vi "Manage logger file txt.vi"(0 "length":i32=1 min=1, 5 "Message to add":string, 11 "error in":errorcluster) -> (15 "error out":errorcluster)   [LabVIEW 2020]
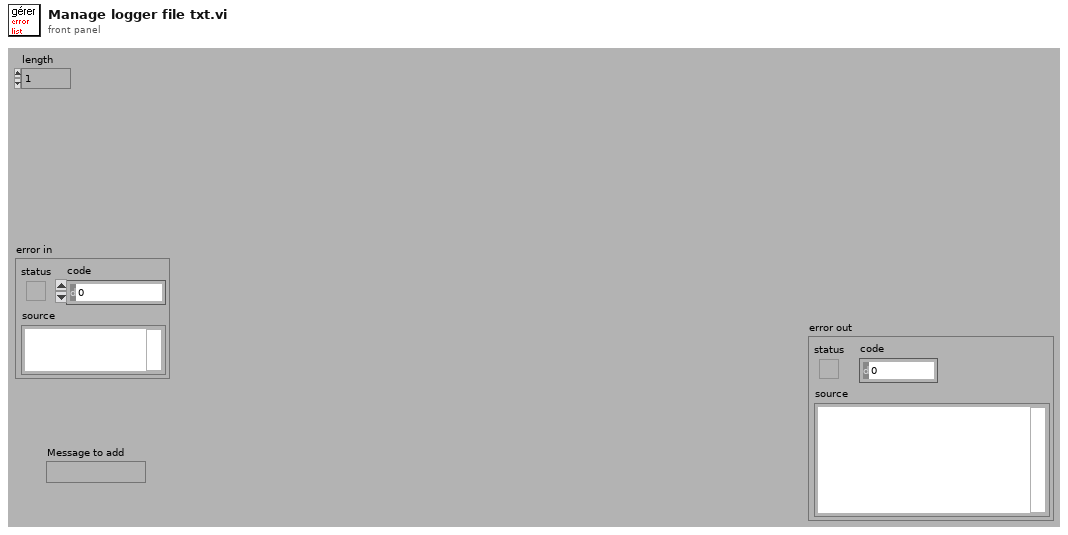
[diagram p1: front panel]
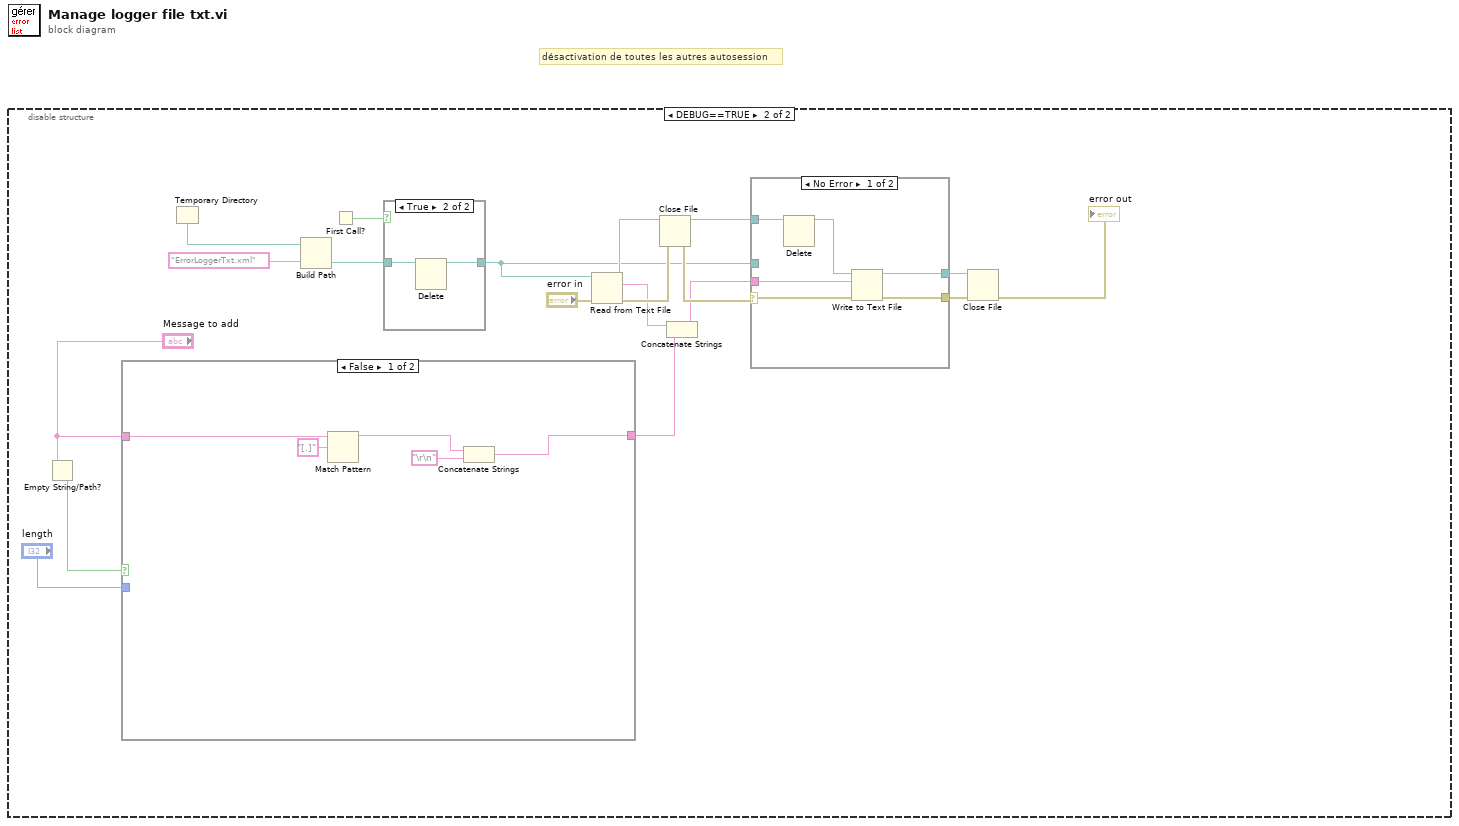
[diagram p0: block diagram]
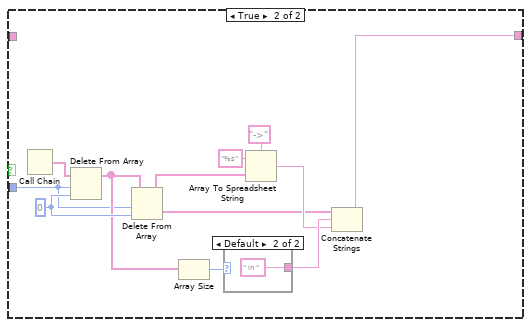
[diagram p3: hidden frame]
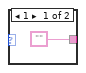
[diagram p4: hidden frame]
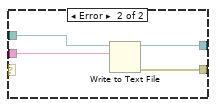
[diagram p6: hidden frame]
diagram:
  # "désactivation de toutes les autres autosession"
  n1 = disable-structure shown="DEBUG==TRUE" {
    frame condition #0 (active) {
    }
    frame condition #1 {
      n2 = Empty String/Path?(string/path="Message to add") -> (empty?=w4:bool)
      n3 = case shown="False" w4 {
        tunnel: [w22 w26] -> w3
        tunnel: "Message to add" -> [w21 _]
        tunnel: "length" -> [_ w25]
        frame False {
          n4 = Match Pattern(string=w21, regular expression="[.]") -> (before substring=w23:string)  [unwired: 1 in, 3 out]
          n5 = Concatenate Strings(w23, "\r\n") -> (w22:string)
        }
        frame True {
          w31 = 0 ("Index")
          n6 = Call Chain() -> (call chain=w36:string[])
          n7 = Delete From Array(array=w36, length=w25, index=w31) -> (array with subset deleted=w27:string[])  [unwired: 1 out]
          n8 = Delete From Array(array=w27, length=w25, index=w31) -> (deleted portion=w28:string[], array with subset deleted=w30:string[])
          n9 = Array Size(array=w27) -> (size(s)=w29:i32)
          n10 = case shown="Default" w29 {
            tunnel: ["" " in " ("Format String")] -> w34
            frame 1 {
            }
            frame Default {
            }
          }
          n11 = Array To Spreadsheet String(delimiter (Tab)="->", array=w30, 3:"%s" ("format string")) -> (spreadsheet string=w33:string)
          n12 = Concatenate Strings(w28, w34, w33) -> (w26:string)
        }
      }
      n13 = Temporary Directory() -> (w19:path)
      n14 = Build Path(base path=w19, name or relative path="ErrorLoggerTxt.xml") -> (appended path=w12:path)
      n15 = First Call?() -> (First Call?: T/F=w14:bool)
      n16 = case shown="True" w14 {
        tunnel: w12 -> [w39 w41]
        tunnel: [w39 w40] -> w13
        frame False {
        }
        frame True {
          n17 = Delete(path (use dialog)=w41) -> (deleted path=w40:path)  [unwired: 4 in, 2 out]
        }
      }
      n18 = Read from Text File(file (use dialog)=w13, error in="error in") -> (refnum out=w15:refnum<file>, text=w6:string, error out=w17:errorcluster)  [unwired: 2 in, 1 out]
      n19 = Close File(refnum=w15, error in=w17) -> (path=w16:path, error out=w18:errorcluster)
      n20 = Concatenate Strings(w6, w3) -> (w7:string)
      n21 = case shown="No Error" w18 {
        selector: w18 -> [w44 _]
        tunnel: w7 -> [w47 w51]
        tunnel: [w46 w50] -> w8
        tunnel: w13 -> [_ w49]
        tunnel: [w45 w48] -> w10
        tunnel: w16 -> [w43 _]
        frame No Error {
          n22 = Delete(path (use dialog)=w43) -> (deleted path=w42:path)  [unwired: 4 in, 2 out]
          n23 = Write to Text File(file (use dialog)=w42, text=w47, error in=w44) -> (refnum out=w46:refnum<file>, error out=w45:errorcluster)  [unwired: 1 in, 1 out]
        }
        frame Error {
          n24 = Write to Text File(file (use dialog)=w49, text=w51) -> (refnum out=w50:refnum<file>, error out=w48:errorcluster)  [unwired: 2 in, 1 out]
        }
      }
      n25 = Close File(refnum=w8, error in=w10) -> (error out=→"error out":errorcluster)  [unwired: 1 out]
    }
  }
